vi "constants.vi"() -> ()   [LabVIEW 2019]
doc: "These global variables store constant values configured in Begin."
panel:
  out "Legal_Shooter_Setpoints":string[](array[string])
  out "Angle_from_LL_to_Horizontal (deg)":dbl
  out "Possible_Shooter_States":string[](array[string])
  out "Height_from_LL_To_Ground_(in)":dbl
  out "Legal_Pipelines":string[](array[string])
  out "Max_Robot_Ground_Speed_(ft/s)":dbl
  out "Legal_Robots":string[](array[string])
  out "Legal_Actuator_Names":string[](array[string])
  out "Possible_Master_States":string[](array[string])
  out "Legal_Auto_Plays":string[](array[string])
  out "Legal_Drivers":string[](array[string])
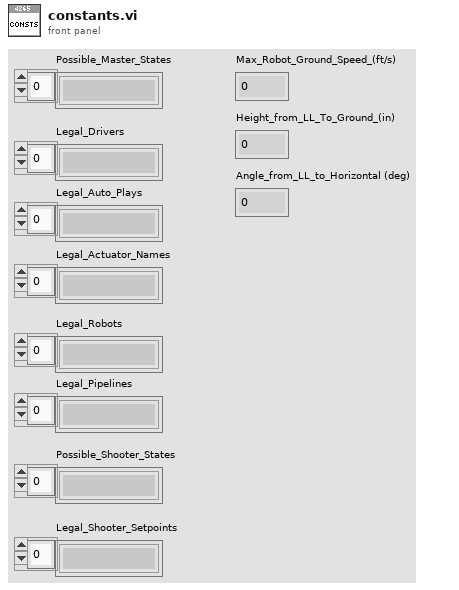
[diagram p1: front panel]
diagram:
